vi "TurnCoordinator.vi"(8 "error in (no error)":errorcluster caption="Fehler (Eingang, kein Fehler)", 10 "MultiWii Data Cluster":T1 {"Altitude abs [m]" format="%.2f"; "Baro T [°C]" format="%.1f"; "Baro P [mbara]" format="%.1f"; "GPS_coord[LON]" format="%#_9f"; "GPS_coord[LAT]" format="%#_9f"; "Altitude [m]" format="%.2f"}) -> (0 "error out":errorcluster caption="Fehler (Ausgang)", 2 "SlipIndicator":T2 scale=-10.0..10.0, 3 "TurnBankPlaneIndicator":picture caption="TurnBankPlanePicture", 4 "RateOfTurn (deg/s)":dbl format="%.2p °/s", 5 "TurnBankStdRate":bool, 6 "BankAngleForStandardRateTurn (deg)":dbl format="%.2f °")   [LabVIEW 2017]
uses:
  SlipIndicator.ctl
  IMU_Functions/IMU_Data_Cluster.ctl
  <vilib>/Utility/miscctls.llb/LVBoundsTypeDef.ctl
  <vilib>/picture/picture.llb/imagedata.ctl
panel:
  in  "Transparent":picture caption="Neue Grafik"
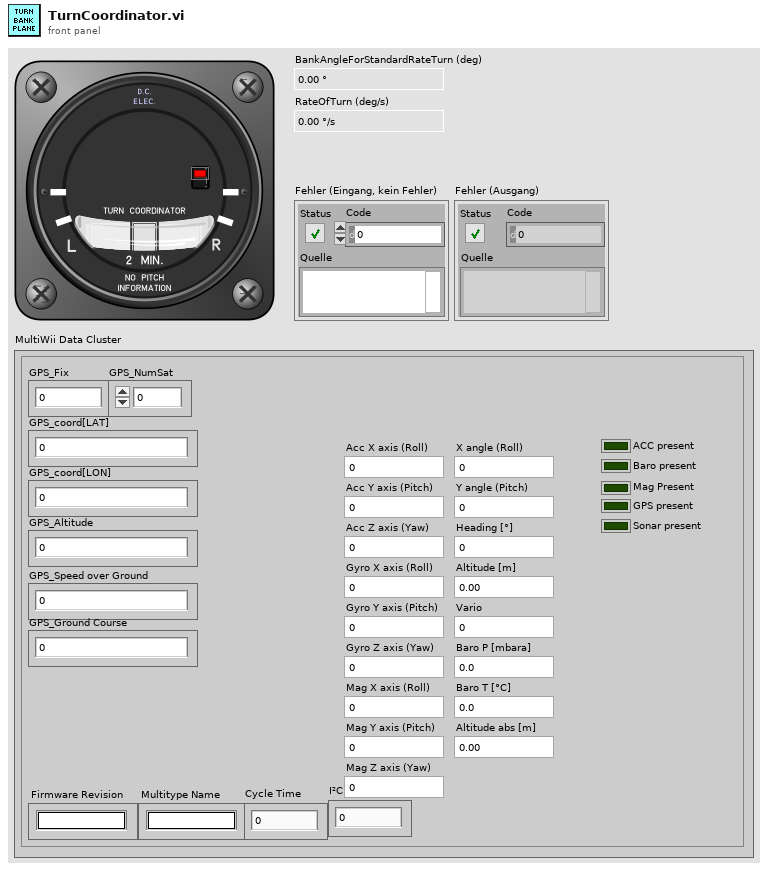
[diagram p1: front panel]
types:
  T1 = typedef "IMU_Data_Cluster.ctl" = cluster{"Firmware Revision":string, "Multitype Name":string, "Cycle Time":u16, "I²C Error Count":u16, "ACC present":bool, "Baro present":bool, "Mag Present":bool, "GPS present":bool, "Sonar present":bool, "Acc X axis (Roll)":dbl, "Acc Y axis (Pitch)":dbl, "Acc Z axis (Yaw)":dbl, "Gyro X axis (Roll)":dbl, "Gyro Y axis (Pitch)":dbl, "Gyro Z axis (Yaw)":dbl, "Mag X axis (Roll)":dbl, "Mag Y axis (Pitch)":dbl, "Mag Z axis (Yaw)":dbl, "X angle (Roll)":dbl, "Y angle (Pitch)":dbl, "Heading [°]":dbl, "Altitude [m]":dbl, "Vario":dbl, "GPS_Fix":u8, "GPS_NumSat":u8, "GPS_coord[LAT]":dbl, "GPS_coord[LON]":dbl, "GPS_Altitude":dbl, "GPS_Speed over Ground":dbl, "GPS_Ground Course":dbl, "Baro P [mbara]":dbl, "Baro T [°C]":dbl, "Altitude abs [m]":dbl}
  T2 = typedef "SlipIndicator.ctl" = dbl
  T3 = typedef "imagedata.ctl" = cluster{"image type":i32, "image depth":i32, "image":u8[], "mask":u8[], "colors":u32[], "Rectangle":cluster{"left":i16, "top":i16, "right":i16, "bottom":i16}}
  T4 = typedef "LVBoundsTypeDef.ctl" = cluster{"Width":u32, "Height":u32}
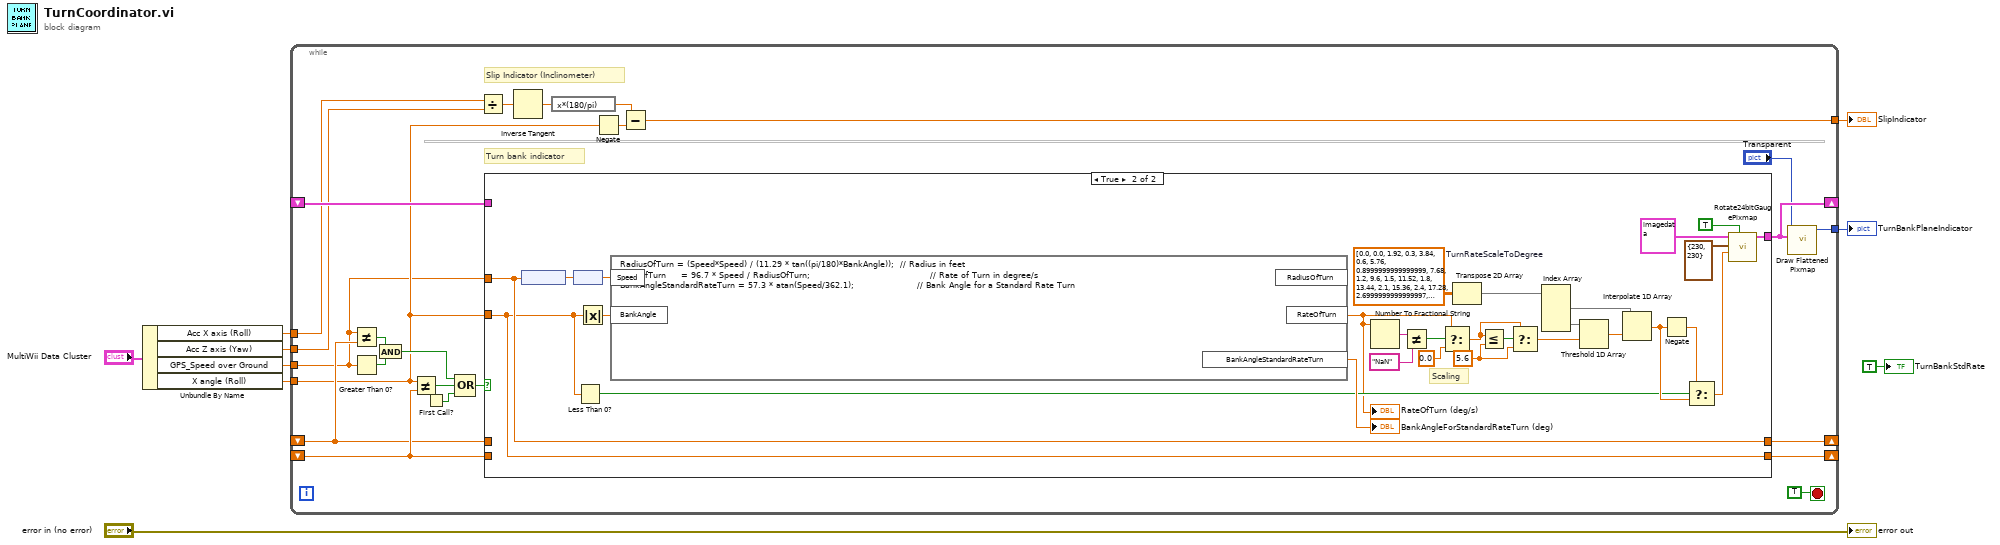
[diagram p0: block diagram]
diagram:
  n1 = Unbundle By Name("MultiWii Data Cluster") -> ("Acc X axis (Roll)"=w5:dbl, "Acc Z axis (Yaw)"=w2:dbl, "GPS_Speed over Ground"=w3:dbl, "X angle (Roll)"=w4:dbl)
  n2 = while {
    shift-right: [w31] -> _
    shift-left: _ -> [w25]
    shift-right: [w30] -> _
    shift-left: _ -> [w29]
    tunnel: [w27] -> w8
    tunnel: w4 -> [w13]
    shift-right: [w23] -> _
    shift-left: _ -> [w22]
    tunnel: [w14] -> w7
    tunnel: w5 -> [w12]
    tunnel: w3 -> [w11]
    tunnel: w2 -> [w10]
    stop <- TRUE stop-if-true
    # "Turn bank indicator"
    # "Slip Indicator (Inclinometer)"
    n3 = Not Equal?(x=w11, y=w22) -> (x != y?=w21:bool)
    n4 = Greater Than 0?(x=w11) -> (x > 0?=w19:bool)
    n5 = And(x=w21, y=w19) -> (x .and. y?=w20:bool)
    n6 = Not Equal?(x=w13, y=w25) -> (x != y?=w32:bool)
    n7 = First Call?() -> (First Call?: T/F=w24:bool)
    n8 = Compound Arithmetic op=OR(w20, w32, w24) -> (w33:bool)
    n9 = Divide(x=w12, y=w10) -> (x/y=w15:dbl)
    n10 = case shown="True" w33 {
      tunnel: [w36 w64] -> w30
      tunnel: w29 -> [w36 _]
      tunnel: w25 -> [w35 _]
      tunnel: [w35 w45] -> w31
      tunnel: w13 -> [_ w45]
      tunnel: w11 -> [_ w61]
      tunnel: [w34 w61] -> w23
      tunnel: w22 -> [w34 _]
      frame False {
      }
      frame True {
        w42 = 5.6 ("y")
        w57 = dbl[][] [[0.0, 0.0], [1.92, 0.3], [3.84, 0.6], [5.76, 0.8999999999999999], [7.68, 1.2], [9.6, 1.5], [11.52, 1.8], [13.44, 2.1], [15.36, 2.4], [17.28, 2.6999999999999997], [19.200000000000003, 2.9999999999999996], [21.120000000000005, 3.2999999999999994], [23.040000000000006, 3.599999999999999], [24.960000000000008, 3.899999999999999], [26.88000000000001, 4.199999999999999], [28.80000000000001, 4.499999999999999], [30.720000000000013, 4.799999999999999], [32.640000000000015, 5.099999999999999], [34.56000000000002, 5.399999999999999], [36.48000000000002, 5.699999999999998]]  # TurnRateScaleToDegree
        # "Scaling"
        n11 = node(w61) -> (w60:dbl[unit])
        n12 = node(w60) -> (w58:dbl)
        n13 = Less Than 0?(x=w45) -> (x < 0?=w46:bool)
        n14 = Absolute Value(x=w45) -> (abs(x)=w59:dbl)
        n15 = formula code="RadiusOfTurn = (Speed*Speed) / (11.29 * tan((pi/180)*BankAngle));  // Radius in feet\nRateOfTurn     = 96.7 * Speed / RadiusOfTurn;                                        // Rate of Turn in degree/s\nBankAngleStandardRateTurn = 57.3 * atan(Speed/362.1);                     // Bank Angle for a Standard Rate Turn"("Speed"=w58, "BankAngle"=w59) -> ("RateOfTurn"=w40:dbl, "BankAngleStandardRateTurn"=→"BankAngleForStandardRateTurn (deg)":dbl)  [unwired: 1 out]
        "RateOfTurn (deg/s)" <- w40
        n16 = Number To Fractional String(number=w40) -> (F-format string=w44:string)  [unwired: 3 in]
        n17 = Not Equal?(x=w44, y="NaN" ("String in F-Format")) -> (x != y?=w41:bool)
        n18 = Select(t=w40, s=w41, f=0.0 ("y")) -> (s? t:f=w39:dbl)
        n19 = Transpose 2D Array(2D array=w57) -> (transposed array=w55:dbl[][])
        n20 = Less Or Equal?(x=w39, y=w42) -> (x <= y?=w48:bool)
        n21 = Select(t=w39, s=w48, f=w42) -> (s? t:f=w47:dbl)
        n22 = Index Array(array=w55) -> (element #1=w53:dbl[], element #2=w54:dbl[])  [unwired: 4 in]
        n23 = Threshold 1D Array(2:w47, 3:w54) -> (0:w56:dbl)  [unwired: 1 in]
        n24 = Interpolate 1D Array(1:w56, 2:w53) -> (0:w51:dbl)
        n25 = Negate(x=w51) -> (-x=w52:dbl)
        n26 = Select(t=w52, s=w46, f=w51) -> (s? t:f=w49:dbl)
        n27 = call "Rotate24bitGaugePixmap.vi"("Maske kombinieren? (F)"=TRUE, "Rotation Angle (degrees)"=w49, "Größe des Darstellungsbereichs"=T4 {"Width"=230, "Height"=230}, "image data"=T3 {"image type"=0, "image depth"=24, "image"=array[158700 elements], "mask"=[], "colors"=[], "Rectangle"={"left"=0, "top"=0, "right"=230, "bottom"=230}}) -> ("image data out"=w64:T3)  [unwired: 7 in]
      }
    }
    n28 = Inverse Tangent(1:w15) -> (0:w16:dbl)
    n29 = expression code="x*(180/pi)"(w16) -> (w17:dbl)
    n30 = Negate(x=w13) -> (-x=w18:dbl)
    n31 = Subtract(x=w17, y=w18) -> (x-y=w14:dbl)
    n32 = call <vilib>:"Draw Flattened Pixmap.vi"("image data"=w30, "picture"="Transparent") -> ("new picture"=w27:picture)  [unwired: 7 out]
  }
  "TurnBankPlaneIndicator" <- w8
  "SlipIndicator" <- w7
  "error out" <- "error in (no error)"
  "TurnBankStdRate" <- TRUE ("TurnBankStdRate")
